vi "Get Page VI.vi"(8 "error in (no error)":errorcluster, 9 "GUID":string, 10 "Item Ref":T1 format="%.0x", 11 "System Explorer Dispatcher Implementation in":refnum<class "System Explorer Dispatcher.lvclass">) -> (0 "error out":errorcluster, 2 "page reference":refnum<vi>, 3 "System Explorer Dispatcher Implementation out":refnum<class "System Explorer Dispatcher.lvclass">)   [LabVIEW 2020, in "AIM ARINC 664 System Explorer.lvlib" / "Implementation.lvlib" / "System Explorer Dispatcher.lvclass"]
uses:
  System Explorer Dispatcher.lvclass
  <vilib>/NI VeriStand/Custom Device API/Custom Device Item Ref.ctl
  System Explorer/Pages/Main Page.vi
  Scripting/Constants.vi
  System Explorer/Pages/Port.vi
  System Explorer/Pages/Tx Generic.vi
  System Explorer/Pages/Logging.vi
  System Explorer/Pages/Secondary Page.vi
  Implementation.lvlib
  Scripting/AIM ARINC 664 Scripting.lvlib
  <vilib>/NI VeriStand/Custom Device API/Custom Device API.lvlib
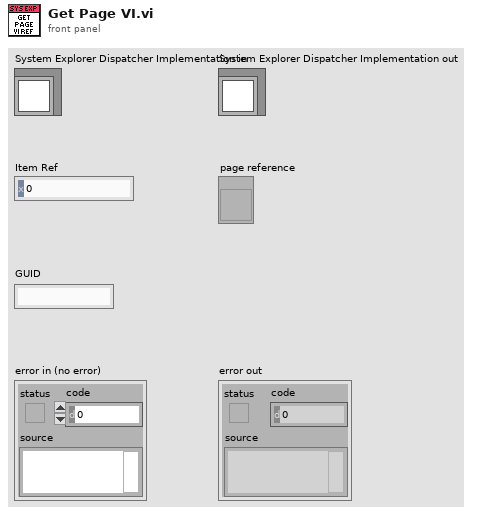
[diagram p1: front panel]
types:
  T1 = typedef "Custom Device API.lvlib/Custom Device Item Ref.ctl" = u64
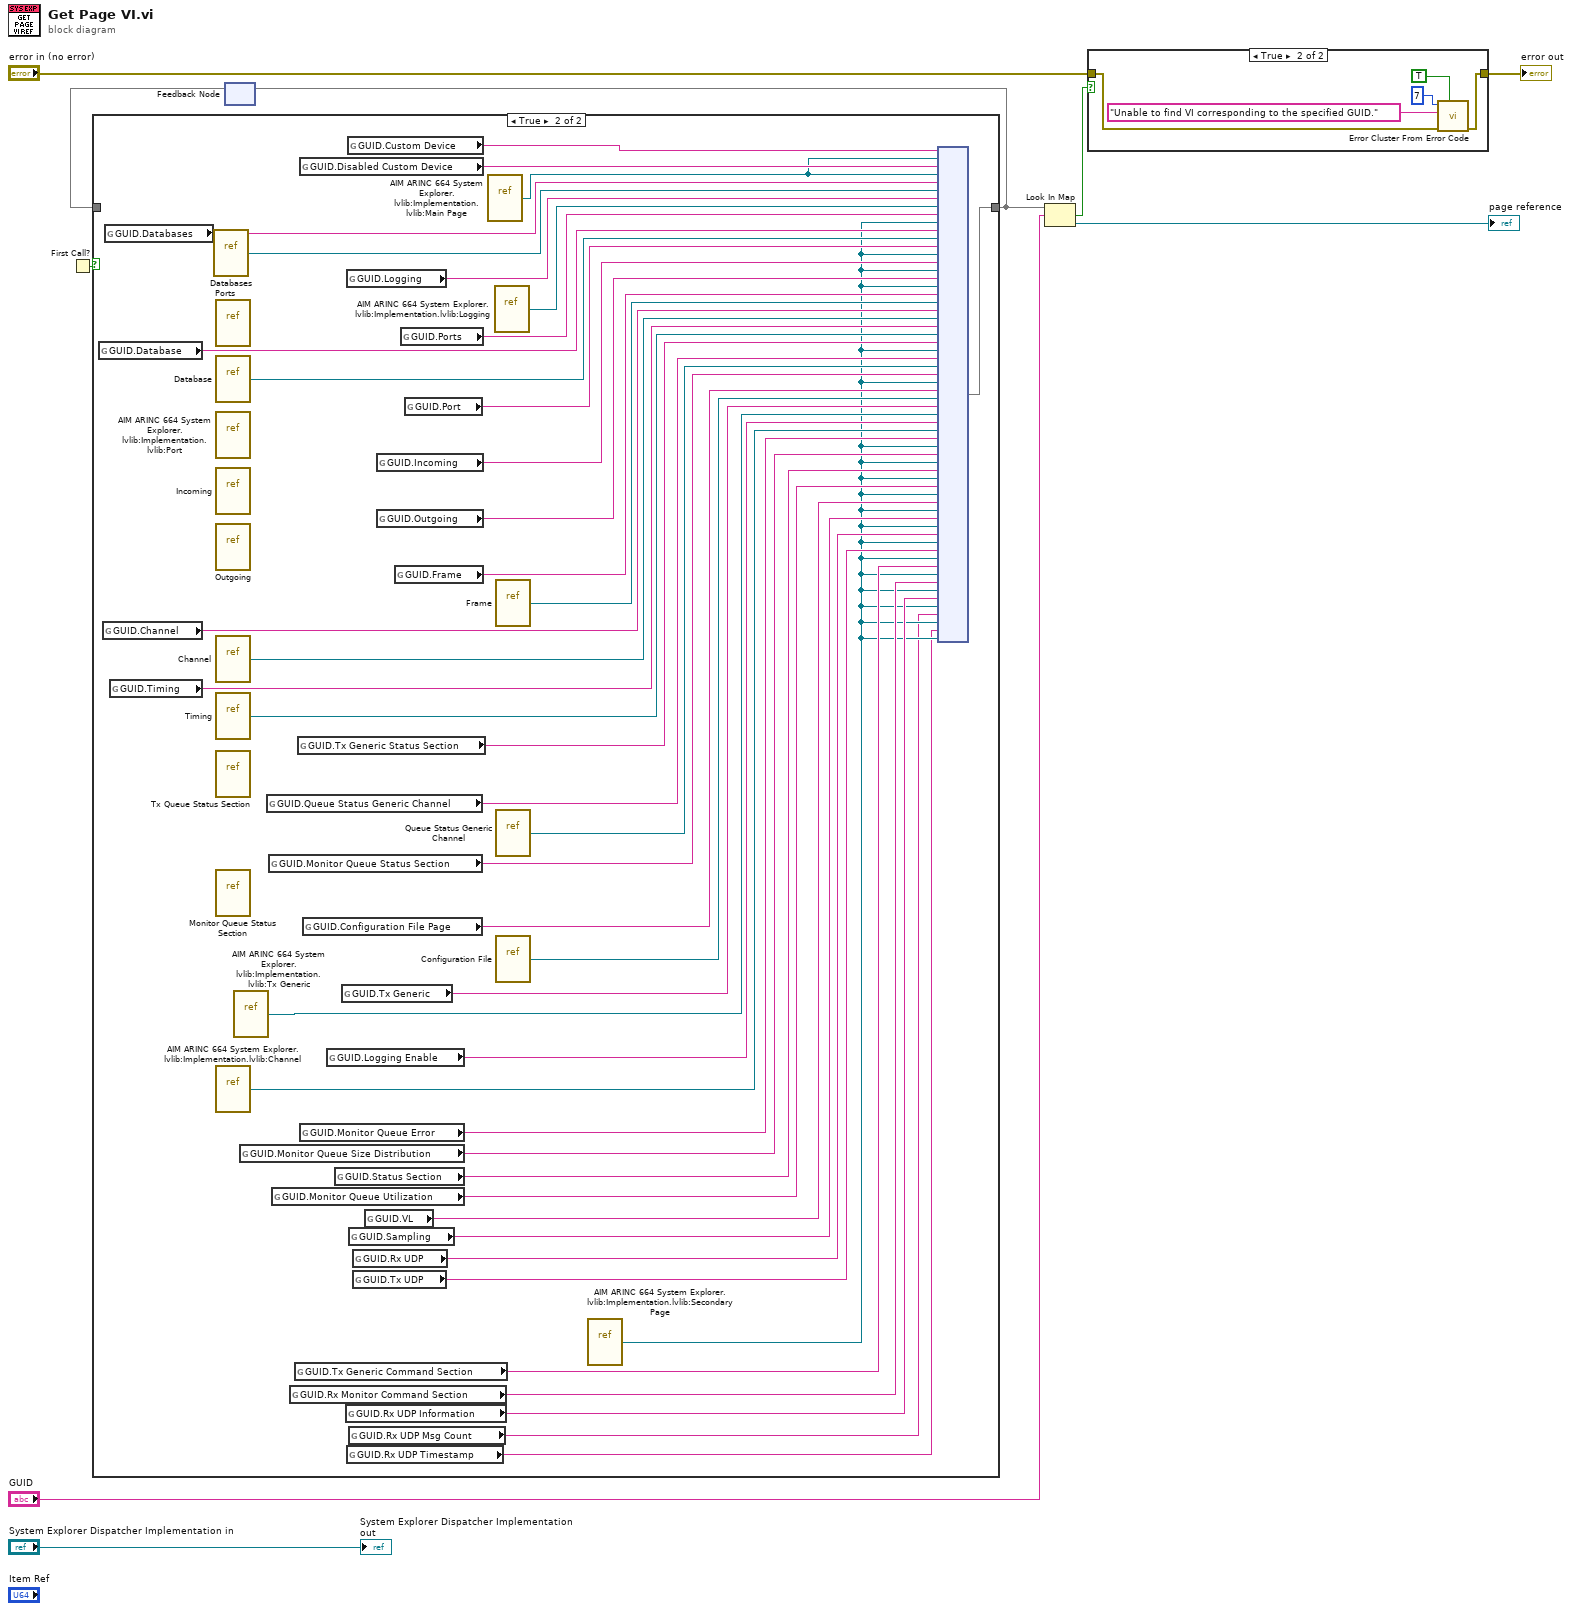
[diagram p0: block diagram]
diagram:
  n1 = First Call?() -> (First Call?: T/F=w8:bool)
  n2 = feedback #1() -> (w7:map{string, refnum<vi>})  [unwired: 1 in]
  n3 = case shown="True" w8 {
    tunnel: [w10 w54] -> w6
    tunnel: w7 -> [w10 _]
    frame False {
    }
    frame True {
      n4 = global read "Constants.vi" "GUID.Database"() -> (w52:string)
      n5 = global read "Constants.vi" "GUID.Channel"() -> (w44:string)
      n6 = global read "Constants.vi" "GUID.Databases"() -> (w32:string)
      n7 = global read "Constants.vi" "GUID.Timing"() -> (w43:string)
      n8 = vi-ref "Databases.vi"() -> (w31:refnum<vi>)
      n9 = vi-ref "Ports.vi"() -> ()  [unwired: 1 out]
      n10 = vi-ref "Database.vi"() -> (w51:refnum<vi>)
      n11 = vi-ref "AIM ARINC 664 System Explorer.lvlib:Implementation.lvlib:Port.vi"() -> ()  [unwired: 1 out]
      n12 = vi-ref "Incoming.vi"() -> ()  [unwired: 1 out]
      n13 = vi-ref "Outgoing.vi"() -> ()  [unwired: 1 out]
      n14 = vi-ref "Channel.vi"() -> (w45:refnum<vi>)
      n15 = vi-ref "Timing.vi"() -> (w42:refnum<vi>)
      n16 = vi-ref "Tx Queue Status Section.vi"() -> ()  [unwired: 1 out]
      n17 = vi-ref "Monitor Queue Status Section.vi"() -> ()  [unwired: 1 out]
      n18 = vi-ref "AIM ARINC 664 System Explorer.lvlib:Implementation.lvlib:Channel.vi"() -> (w27:refnum<vi>)
      n19 = vi-ref "AIM ARINC 664 System Explorer.lvlib:Implementation.lvlib:Tx Generic.vi"() -> (w15:refnum<vi>)
      n20 = global read "Constants.vi" "GUID.Monitor Queue Size Distribution"() -> (w25:string)
      n21 = global read "Constants.vi" "GUID.Queue Status Generic Channel"() -> (w40:string)
      n22 = global read "Constants.vi" "GUID.Monitor Queue Status Section"() -> (w38:string)
      n23 = global read "Constants.vi" "GUID.Monitor Queue Utilization"() -> (w23:string)
      n24 = global read "Constants.vi" "GUID.Rx Monitor Command Section"() -> (w16:string)
      n25 = global read "Constants.vi" "GUID.Tx Generic Command Section"() -> (w17:string)
      n26 = global read "Constants.vi" "GUID.Tx Generic Status Section"() -> (w41:string)
      n27 = global read "Constants.vi" "GUID.Disabled Custom Device"() -> (w33:string)
      n28 = global read "Constants.vi" "GUID.Monitor Queue Error"() -> (w26:string)
      n29 = global read "Constants.vi" "GUID.Configuration File Page"() -> (w37:string)
      n30 = global read "Constants.vi" "GUID.Logging Enable"() -> (w28:string)
      n31 = global read "Constants.vi" "GUID.Status Section"() -> (w24:string)
      n32 = global read "Constants.vi" "GUID.Tx Generic"() -> (w35:string)
      n33 = global read "Constants.vi" "GUID.Rx UDP Information"() -> (w14:string)
      n34 = global read "Constants.vi" "GUID.Logging"() -> (w29:string)
      n35 = global read "Constants.vi" "GUID.Rx UDP Timestamp"() -> (w11:string)
      n36 = global read "Constants.vi" "GUID.Custom Device"() -> (w34:string)
      n37 = global read "Constants.vi" "GUID.Sampling"() -> (w20:string)
      n38 = global read "Constants.vi" "GUID.Rx UDP Msg Count"() -> (w12:string)
      n39 = global read "Constants.vi" "GUID.Rx UDP"() -> (w19:string)
      n40 = global read "Constants.vi" "GUID.Tx UDP"() -> (w18:string)
      n41 = global read "Constants.vi" "GUID.VL"() -> (w21:string)
      n42 = global read "Constants.vi" "GUID.Incoming"() -> (w49:string)
      n43 = global read "Constants.vi" "GUID.Outgoing"() -> (w48:string)
      n44 = global read "Constants.vi" "GUID.Frame"() -> (w47:string)
      n45 = global read "Constants.vi" "GUID.Ports"() -> (w53:string)
      n46 = global read "Constants.vi" "GUID.Port"() -> (w50:string)
      n47 = vi-ref "AIM ARINC 664 System Explorer.lvlib:Implementation.lvlib:Main Page.vi"() -> (w22:refnum<vi>)
      n48 = vi-ref "AIM ARINC 664 System Explorer.lvlib:Implementation.lvlib:Logging.vi"() -> (w30:refnum<vi>)
      n49 = vi-ref "Frame.vi"() -> (w46:refnum<vi>)
      n50 = vi-ref "Queue Status Generic Channel.vi"() -> (w39:refnum<vi>)
      n51 = vi-ref "Configuration File.vi"() -> (w36:refnum<vi>)
      n52 = vi-ref "AIM ARINC 664 System Explorer.lvlib:Implementation.lvlib:Secondary Page.vi"() -> (w13:refnum<vi>)
      n53 = node(w34, w22, w33, w22, w32, w31, w29, w30, w53, w13, w52, w51, w50, w13, w49, w13, w48, w13, w47, w46, w44, w45, w43, w42, w41, w13, w40, w39, w38, w13, w37, w36, w35, w15, w28, w27, w26, w13, w25, w13, w24, w13, w23, w13, w21, w13, w20, w13, w19, w13, w18, w13, w17, w13, w16, w13, w14, w13, w12, w13, w11, w13) -> (w54:map{string, refnum<vi>})
    }
  }
  n54 = feedback-in #1(w6) -> ()
  n55 = Look In Map(map=w6, key="GUID") -> (key not found?=w4:bool, value=→"page reference":refnum<vi>)  [unwired: 1 in]
  n56 = case shown="True" w4 {
    tunnel: [w55 w57] -> w3
    tunnel: "error in (no error)" -> [w55 w56]
    frame False {
    }
    frame True {
      n57 = call <vilib>:"Error Cluster From Error Code.vi"("show call chain? (False)"=TRUE, "error in (no error)"=w56, "error message (\"\")"="Unable to find VI corresponding to the specified GUID." ("error message (\"\")"), "error code (0)"=7) -> ("error out"=w57:errorcluster)  [unwired: 5 in]
    }
  }
  "error out" <- w3
  "System Explorer Dispatcher Implementation out" <- "System Explorer Dispatcher Implementation in"
